vi "AddTestMethod_CreateNewWizard_Invoke.vi"(10 "Cluster":T1, 11 "Wizard":T2) -> (3 "Canceled":bool)   [LabVIEW 2013]
uses:
  <resource>/Framework/Providers/API/ItemRef.ctl
  <resource>/Framework/Providers/API/mxLvNIIM.ctl
  Scripter/Scripter.lvlib
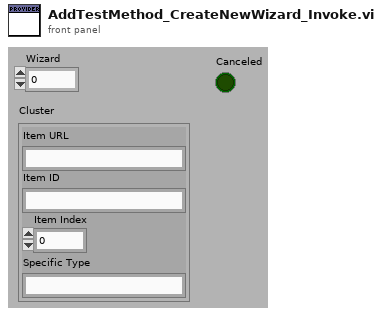
[diagram p1: front panel]
types:
  T1 = typedef "mxLvNIIM.ctl" = cluster{"Item URL":string, "Item ID":string, "Item Index":i32, "Specific Type":string}
  T2 = typedef "ItemRef.ctl" = u64
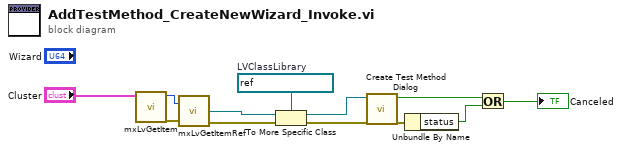
[diagram p0: block diagram]
diagram:
  w7 = refnum<vi> refnum  # LVClassLibrary
  n1 = call <resource>:"mxLvGetItem.vi"("NIIM"="Cluster") -> ("error out"=w10:errorcluster, "Item"=w11:T2)  [unwired: 9 in]
  n2 = call <resource>:"mxLvGetItemRef.vi"("Item"=w11, "error in"=w10) -> ("Item Refnum"=w8:refnum<vi>, "error out"=w9:errorcluster)  [unwired: 1 out]
  n3 = To More Specific Class(target class=w7, reference=w8, error in=w9) -> (specific class reference=w5:refnum<vi>, error out=w6:errorcluster)
  n4 = call "Create Test Method Dialog.vi"("Error In"=w6, "Class Ref"=w5) -> ("Error Out"=w2:errorcluster, "Cancelled?"=w4:bool)  [unwired: 8 in]
  n5 = Unbundle By Name(w2) -> ("status"=w1:bool)
  n6 = Or(x=w4, y=w1) -> (x .or. y?=→"Canceled":bool)
